vi "Initialize From Settings.vi"(8 "error in (no error)":errorcluster, 10 "settings":cluster{"key":string, "value":string}[](array[cluster]), 11 "Transfer Configuration in":refnum<class "Transfer Configuration.lvclass">) -> (0 "error out":errorcluster, 3 "Transfer Configuration out":refnum<class "Transfer Configuration.lvclass">)   [LabVIEW 2017, in "PXImc.lvlib" / "Transfer Configuration.lvclass"]
uses:
  Transfer Configuration.lvclass
  Transfer Configuration.lvclass/Transfer Configuration.ctl
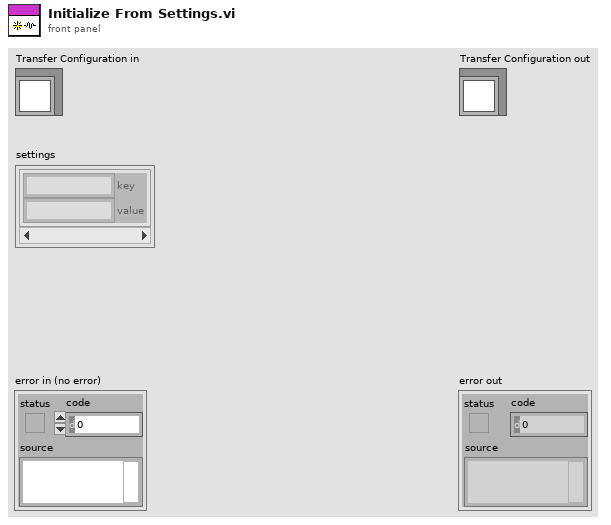
[diagram p1: front panel]
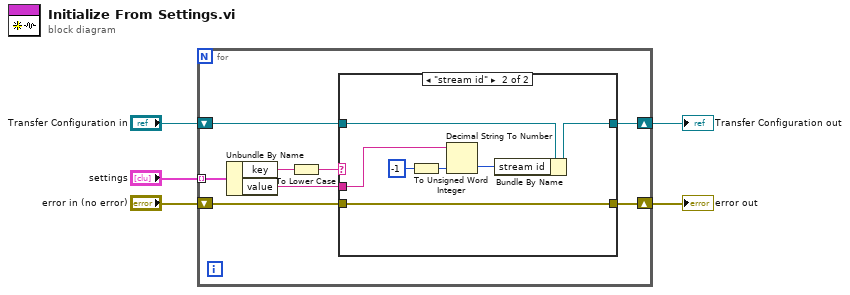
[diagram p0: block diagram]
diagram:
  n1 = for {
    tunnel: "settings" -> [w13] mode=indexing
    shift-right: [w6] -> w4
    shift-left: "error in (no error)" -> [w9]
    shift-right: [w7] -> w2
    shift-left: "Transfer Configuration in" -> [w8]
    n2 = Unbundle By Name(w13) -> ("key"=w12:string, "value"=w10:string)
    n3 = To Lower Case(string=w12) -> (all lower case string=w11:string)
    n4 = case shown="\"stream id\"" w11 {
      tunnel: w10 -> [_ w22]
      tunnel: w9 -> [w14 w16]
      tunnel: w8 -> [w15 w18]
      tunnel: [w15 w17] -> w7
      tunnel: [w14 w16] -> w6
      frame Default {
        # "Unknown setting."
      }
      frame "stream id" {
        n5 = To Unsigned Word Integer(number=i16 -1 ("default (0 I32)")) -> (unsigned 16bit integer=w20:u16)
        n6 = Decimal String To Number(string=w22, default (0L)=w20) -> (number=w19:u16)  [unwired: 1 in, 1 out]
        n7 = Bundle By Name(cluster=w18, "stream id"=w19) -> (w17:refnum<class "Transfer Configuration.lvclass">)
      }
    }
  }
  "error out" <- w4
  "Transfer Configuration out" <- w2
